vi "Minimum Code To Run.Vi"   [LabVIEW 2013]
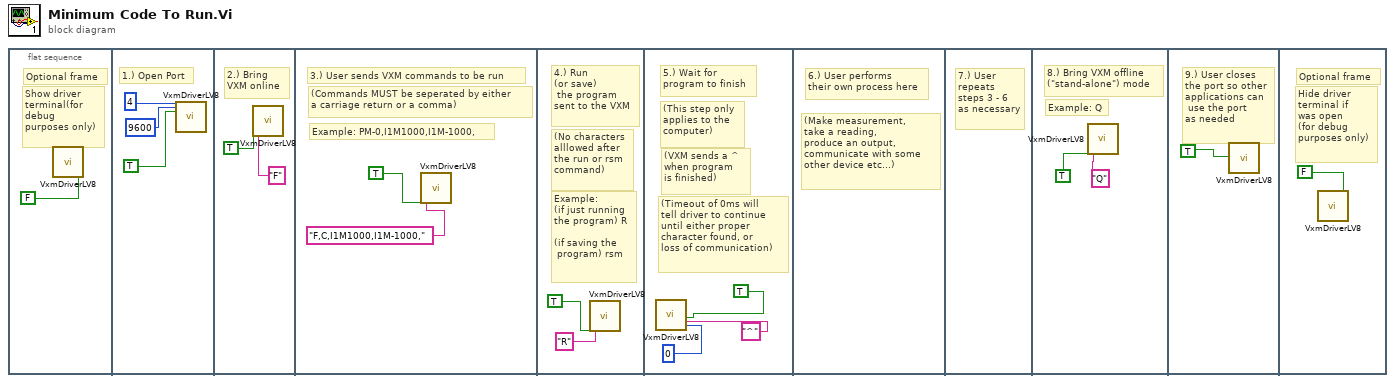
[diagram p0: block diagram]
diagram:
  n1 = flat-sequence {
    frame #0 {
      # "Show driver\nterminal(for\ndebug \npurposes only)"
      # "Optional frame"
      n2 = call "VxmDriverLV8.vi"("Show Terminal"=FALSE) -> ()  [unwired: 21 in, 6 out]
    }
    frame #1 {
      # "1.) Open Port"
      n3 = call "VxmDriverLV8.vi"("Port"=4, "Baud Rate"=9600, "Open Port"=TRUE) -> ()  [unwired: 19 in, 6 out]
    }
    frame #2 {
      # "2.) Bring\nVXM online"
      n4 = call "VxmDriverLV8.vi"("Send\nchars\nto port"=TRUE, "Chars to send"="F") -> ()  [unwired: 20 in, 6 out]
    }
    frame #3 {
      # "(Commands MUST be seperated by either\na carriage return or a comma)"
      # "Example: PM-0,I1M1000,I1M-1000,"
      # "3.) User sends VXM commands to be run"
      n5 = call "VxmDriverLV8.vi"("Send\nchars\nto port"=TRUE, "Chars to send"="F,C,I1M1000,I1M-1000,") -> ()  [unwired: 20 in, 6 out]
    }
    frame #4 {
      # "Example:\n(if just running \nthe program) R\n\n(if saving the\n program) rsm"
      # "(No characters\nalllowed after \nthe run or rsm \ncommand)"
      # "4.) Run \n(or save)\n the program \nsent to the VXM"
      n6 = call "VxmDriverLV8.vi"("Send\nchars\nto port"=TRUE, "Chars to send"="R") -> ()  [unwired: 20 in, 6 out]
    }
    frame #5 {
      # "(Timeout of 0ms will\ntell driver to continue\nuntil either proper \ncharacter found, or\nloss of communication)"
      # "(VXM sends a ^ \nwhen program \nis finished)"
      # "(This step only \napplies to the \ncomputer)"
      # "5.) Wait for \nprogram to finish"
      n7 = call "VxmDriverLV8.vi"("Wait\nfor \nchar"=TRUE, "Char(s) to wait for"="^", "Char\nTimeout\nTime (ms)"=0) -> ()  [unwired: 19 in, 6 out]
    }
    frame #6 {
      # "(Make measurement,\ntake a reading,\nproduce an output, \ncommunicate with some \nother device etc...)"
      # "6.) User performs \ntheir own process here"
    }
    frame #7 {
      # "7.) User\nrepeats \nsteps 3 - 6\nas necessary"
    }
    frame #8 {
      # "Example: Q"
      # "8.) Bring VXM offline \n(\"stand-alone\") mode"
      n8 = call "VxmDriverLV8.vi"("Send\nchars\nto port"=TRUE, "Chars to send"="Q") -> ()  [unwired: 20 in, 6 out]
    }
    frame #9 {
      # "9.) User closes\nthe port so other\napplications can\n use the port\nas needed"
      n9 = call "VxmDriverLV8.vi"("Close Port"=TRUE) -> ()  [unwired: 21 in, 6 out]
    }
    frame #10 {
      # "Hide driver\nterminal if\nwas open\n(for debug \npurposes only)"
      # "Optional frame"
      n10 = call "VxmDriverLV8.vi"("Hide Terminal"=FALSE) -> ()  [unwired: 21 in, 6 out]
    }
  }
